vi "Read Acknowledgement.vi"(8 "error in (no error)":errorcluster, 11 "VISA resource name":refnum<visa-resource-name>) -> (0 "error out":errorcluster, 3 "VISA resource name out":refnum<visa-resource-name>)   [LabVIEW 2014, in "Associated Research SC6540.lvlib"]
doc: "Reads the response from the instrument, when it is connected in serial mode (This is because the instrument sends the ACK or NACK automatically in this mode of communication)\n\nThis is a Private type VI and meant for getting the acknowledgement alone."
uses:
  <instrlib>/Associated Research SC6540/Associated Research SC6540.lvlib
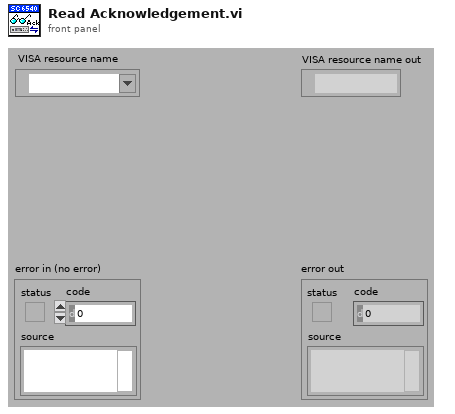
[diagram p1: front panel]
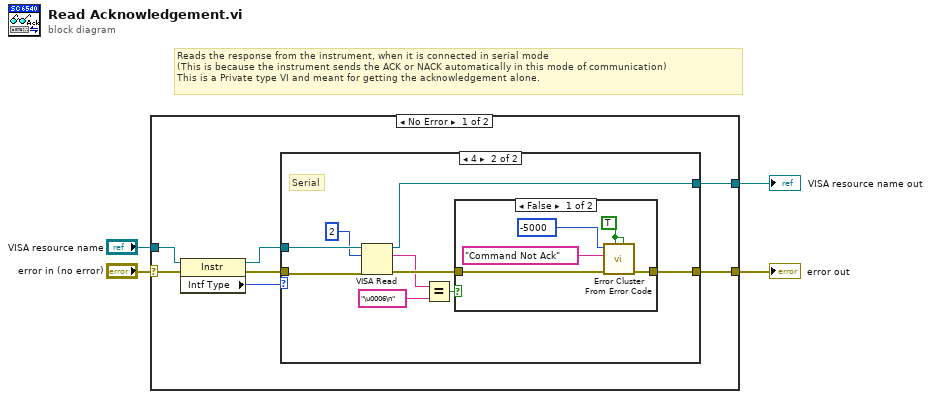
[diagram p0: block diagram]
diagram:
  # "Reads the response from the instrument, when it is connected in serial mode \n(This is because the instrument sends the ACK or NACK automatically in this mode of communication)\nThis is a Private type VI and meant for getting the acknowledgement alone."
  n1 = case shown="No Error" "error in (no error)" {
    selector: "error in (no error)" -> [w7 w30]
    tunnel: "VISA resource name" -> [w8 w29]
    tunnel: [w6 w29] -> w2
    tunnel: [w5 w30] -> w1
    frame No Error {
      n2 = property on="Property Node" class="Instr"(reference=w8, error in=w7) -> (reference out=w10:refnum<visa-resource-name>, error out=w11:errorcluster, "Intf Type"=w9:u16)
      n3 = case shown="4" w9 {
        tunnel: w10 -> [w13 w15]
        tunnel: [w13 w19] -> w6
        tunnel: w11 -> [w12 w16]
        tunnel: [w12 w21] -> w5
        frame 1, Default {
          # "GPIB, Ethernet"
        }
        frame 4 {
          # "Serial"
          n4 = VISA Read(VISA resource name=w15, byte count=u32 2, error in (no error)=w16) -> (VISA resource name out=w19:refnum<visa-resource-name>, read buffer=w17:string, error out=w22:errorcluster)  [unwired: 1 out]
          n5 = Equal?(x=w17, y="\u0006\n") -> (x = y?=w18:bool)
          n6 = case shown="False" w18 {
            tunnel: w22 -> [w27 w28]
            tunnel: [w26 w28] -> w21
            frame False {
              w25 = TRUE ("show call chain? (False)")
              n7 = call <vilib>:"Error Cluster From Error Code.vi"("is warning? (False)"=w25, "show call chain? (False)"=w25, "error in (no error)"=w27, "error message (\"\")"="Command Not Ack" ("error message (\"\")"), "error code (0)"=-5000) -> ("error out"=w26:errorcluster)  [unwired: 4 in]
            }
            frame True {
            }
          }
        }
      }
    }
    frame Error {
    }
  }
  "VISA resource name out" <- w2
  "error out" <- w1
